vi "record track.vi"(6 "index":i32, 7 "Record":bool, 9 "AudioIn/Right (N Samples)":dbl[](array[numeric]), 10 "AudioIn/Left (N Samples)":dbl[](array[numeric]), 11 "Track In":T1) -> (3 "Track Out":T1)   [LabVIEW 2014]
uses:
  Controls/Audio In.ctl
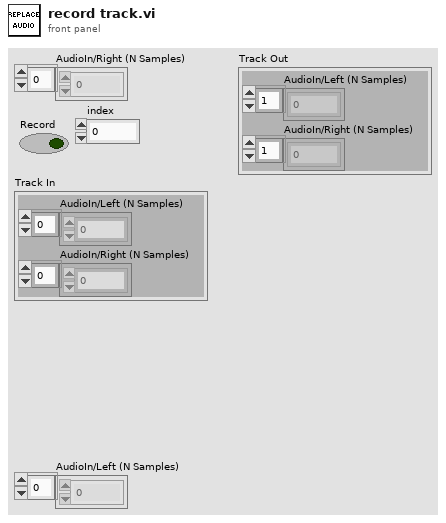
[diagram p1: front panel]
types:
  T1 = typedef "Audio In.ctl" = cluster{"AudioIn/Left (N Samples)":dbl[], "AudioIn/Right (N Samples)":dbl[]}
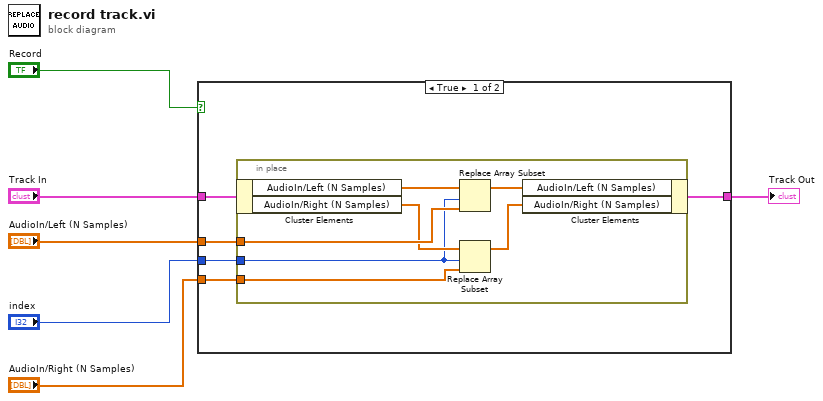
[diagram p0: block diagram]
diagram:
  n1 = case shown="True" "Record" {
    tunnel: "Track In" -> [w10 w19]
    tunnel: "AudioIn/Left (N Samples)" -> [w11 _]
    tunnel: "AudioIn/Right (N Samples)" -> [w9 _]
    tunnel: [w8 w19] -> w6
    tunnel: "index" -> [w7 _]
    frame True {
      n2 = in-place {
        in-place-border: w11 -> [w17]
        in-place-border: w9 -> [w13]
        in-place-border: w7 -> [w14]
        n3 = in-place-cluster #1(w10) -> ("AudioIn/Left (N Samples)"=w18:dbl[], "AudioIn/Right (N Samples)"=w15:dbl[])
        n4 = Replace Array Subset(array=w18, new element=w17, index=w14) -> (w16:dbl[])
        n5 = Replace Array Subset(array=w15, new element=w13, index=w14) -> (w12:dbl[])
        n6 = in-place-cluster #1("AudioIn/Left (N Samples)"=w16, "AudioIn/Right (N Samples)"=w12) -> (w8:T1)
      }
    }
    frame False {
    }
  }
  "Track Out" <- w6
